vi "MoveTest.vi"() -> ()   [LabVIEW 2010]
panel:
  out "Complete?":bool
  in  "stop":bool
  out "error out":errorcluster
  in  "Serial":i32=83830377
  in  "MG17Motor":refnum<k7>(container)
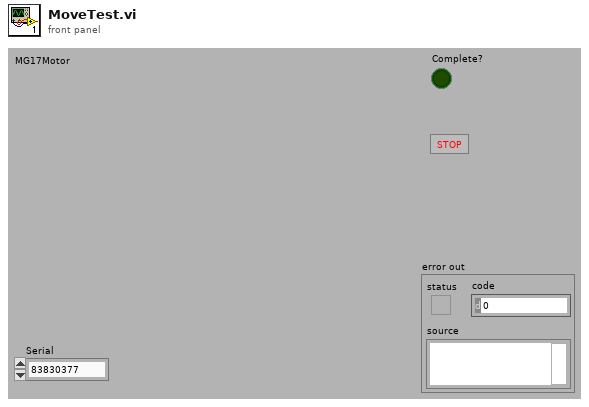
[diagram p1: front panel]
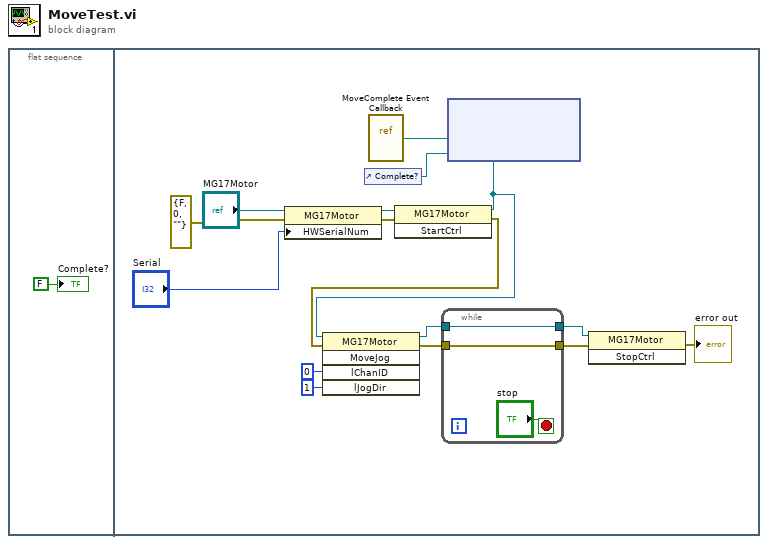
[diagram p0: block diagram]
diagram:
  n1 = flat-sequence {
    frame #0 {
      "Complete?" <- FALSE ("Complete?")
    }
    frame #1 {
      n2 = property class="MG17Motor"(reference="MG17Motor", error in=errorcluster {"status"=FALSE, "code"=0, "source"=""} ("error in (no error)"), "HWSerialNum"="Serial") -> (reference out=w16:refnum<k7>, error out=w15:errorcluster)
      n3 = control-ref of="Complete?"() -> (w3:refnum<vi>)
      n4 = vi-ref "MoveComplete Event Callback.vi"() -> ("vi reference"=w2:refnum<vi>)
      n5 = invoke class="MG17Motor" method="StartCtrl"(reference=w16, error in=w15) -> (reference out=w9:refnum<k7>, error out=w8:errorcluster)  [unwired: 1 in, 1 out]
      n6 = invoke class="MG17Motor" method="MoveJog"(reference=w9, error in=w8, "lChanID"=0, "lJogDir"=1) -> (reference out=w7:refnum<k7>, error out=w6:errorcluster)  [unwired: 1 in, 3 out]
      n7 = while {
        tunnel: w7 -> [w18]
        tunnel: w6 -> [w19]
        tunnel: [w19] -> w5
        tunnel: [w18] -> w4
        stop <- "stop" stop-if-true
      }
      n8 = node(w9, w2, w3) -> ()  [unwired: 2 in, 2 out]
      n9 = invoke class="MG17Motor" method="StopCtrl"(reference=w4, error in=w5) -> (error out=→"error out":errorcluster)  [unwired: 1 in, 2 out]
    }
  }
